vi "Update Motor Config Control Settings.vi"(8 "error in (no error)":errorcluster, 10 "Motor Config Data":T1[](array[typedef]), 11 "Motor Config Refs":refnum<vi>[](array[refnum])) -> (0 "error out":errorcluster)   [LabVIEW 2018]
uses:
  Ctls/MotorConfig.ctl
  Ctls/MotroConfigData.ctl
  Ctls/MagType.ctl
panel:
  in  "电机2配置":T2
  in  "电机1配置":T2
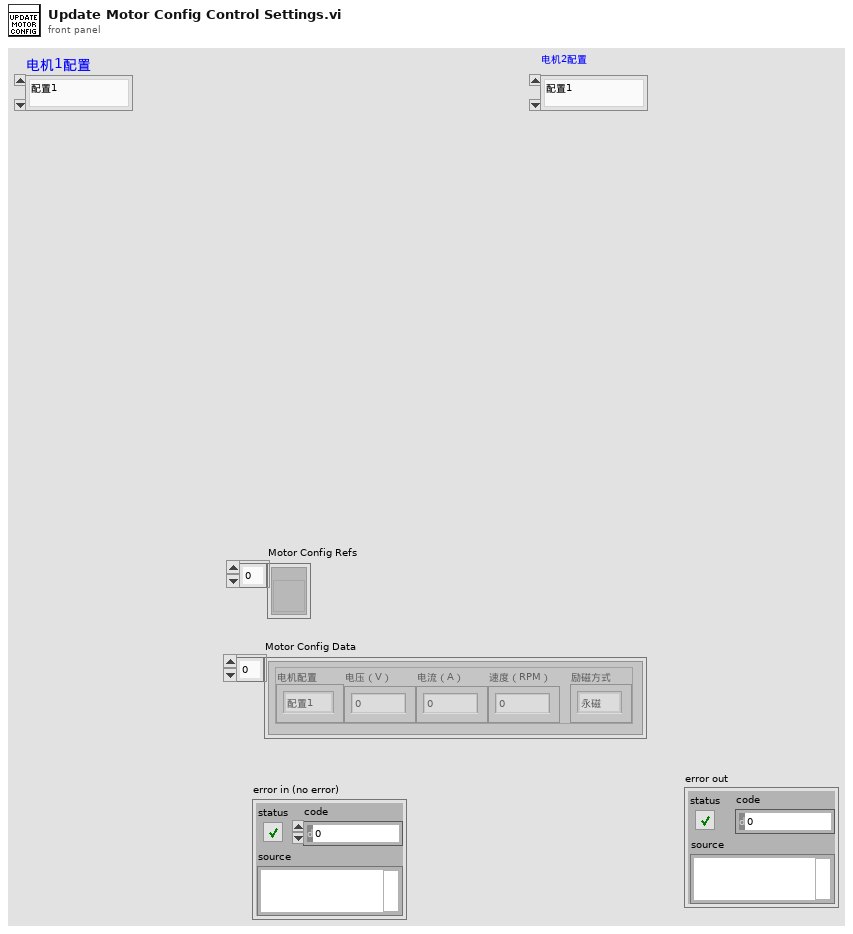
[diagram p1: front panel]
types:
  T1 = typedef "MotroConfigData.ctl" = cluster{"电机配置":T2, "电压（V）":dbl, "电流（A）":dbl, "速度（RPM）":dbl, "励磁方式":T3}
  T2 = typedef "MotorConfig.ctl" = enum16{"配置1", "配置2", "配置3", "配置4"}
  T3 = typedef "MagType.ctl" = enum16{"永磁", "励磁"}
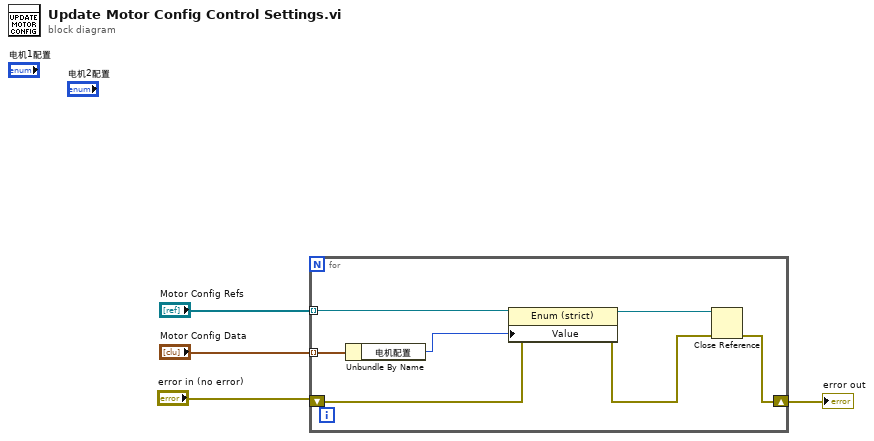
[diagram p0: block diagram]
diagram:
  n1 = for {
    tunnel: "Motor Config Refs" -> [w7] mode=indexing
    tunnel: "Motor Config Data" -> [w9] mode=indexing
    shift-right: [w5] -> w1
    shift-left: "error in (no error)" -> [w11]
    n2 = Unbundle By Name(w9) -> ("电机配置"=w8:T2)
    n3 = property class="Enum (strict)"(reference=w7, error in=w11, "Value"=w8) -> (reference out=w10:refnum<vi>, error out=w6:errorcluster)
    n4 = Close Reference(reference=w10, error in (no error)=w6) -> (error out=w5:errorcluster)
  }
  "error out" <- w1
